vi "cancellable wait func.vi"(10 "task token":refnum<class "null task token.lvclass">, 11 "parameters":variant) -> (1 "error":errorcluster, 2 "data":variant, 3 "data ID":string)   [LabVIEW 2013]
uses:
  task token/null task token.lvclass
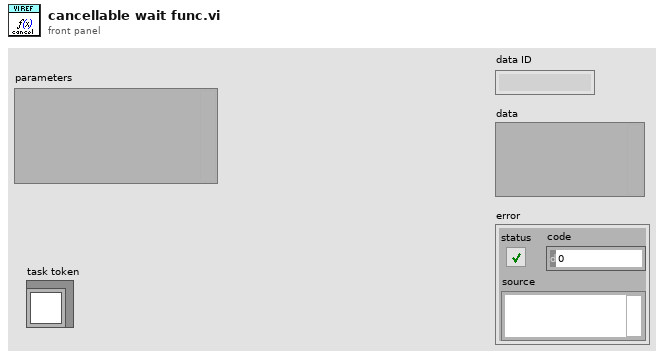
[diagram p1: front panel]
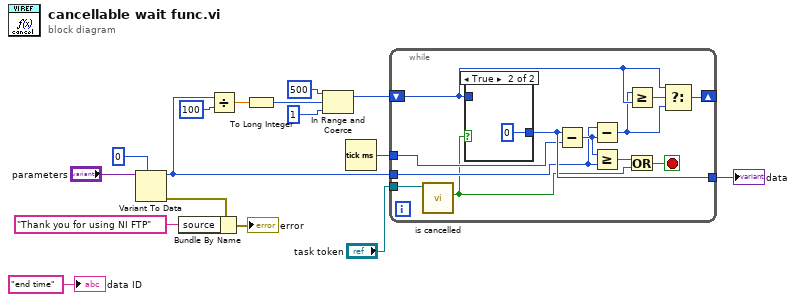
[diagram p0: block diagram]
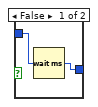
[diagram p2: hidden frame]
diagram:
  n1 = Variant To Data(type=u32 0 ("milliseconds to wait"), Variant="parameters") -> (data=w6:u32, error out=w15:errorcluster)  [unwired: 1 in]
  n2 = Bundle By Name(cluster=w15, "source"="Thank you for using NI FTP") -> (→"error":errorcluster)
  n3 = Divide(x=w6, y=u32 100) -> (x/y=w11:dbl)
  n4 = To Long Integer(number=w11) -> (32bit integer=w10:i32)
  n5 = In Range and Coerce(upper limit=500, x=w10, lower limit=1) -> (coerced(x)=w7:i32)  [unwired: 1 out]
  n6 = Tick Count (ms)() -> (millisecond timer value=w13:u32)
  n7 = while {
    tunnel: [w27] -> w1
    tunnel: "task token" -> [w28]
    tunnel: w13 -> [w26]
    tunnel: w6 -> [w22]
    shift-right: [w19] -> _
    shift-left: w7 -> [w20]
    stop <- w25 stop-if-true
    n8 = call-dynamic "is cancelled.vi"("null task token in"=w28) -> ("cancelled?"=w17:bool)  [unwired: 9 in, 1 out]
    n9 = case shown="True" w17 {
      tunnel: [w30 u32 0 ("millisecond timer value")] -> w27
      tunnel: w20 -> [w29 _]
      frame False {
        n10 = Wait (ms)(milliseconds to wait=w29) -> (millisecond timer value=w30:u32)
      }
      frame True {
      }
    }
    n11 = Subtract(x=w27, y=w26) -> (x-y=w23:u32)
    n12 = Subtract(x=w22, y=w23) -> (x-y=w18:u32)
    n13 = Greater Or Equal?(x=w23, y=w22) -> (x >= y?=w24:bool)
    n14 = Greater Or Equal?(x=w18, y=w20) -> (x >= y?=w21:bool)
    n15 = Or(x=w24, y=w17) -> (x .or. y?=w25:bool)
    n16 = Select(t=w20, s=w21, f=w18) -> (s? t:f=w19:u32)
  }
  "data" <- w1
  "data ID" <- "end time" ("data ID")
